vi "FTW-SyncServer-Reply.vi"(0 "FTW Synchronous Server":refnum<data-value>, 5 "Response":string, 7 "Send Timeout":i32 format="%dmsec", 11 "error in":errorcluster) -> (4 "FTW Synchronous Server out":refnum<data-value>, 15 "error out":errorcluster)   [LabVIEW 2014]
uses:
  core/FTW-SyncServer-Core-Type.ctl
  error/FTW-ERR-ThrowGenericError.vi
  error/FTW-ERR-ThrowError.vi
  error/FTW-ERR-CallChain.vi
  string/FTW-STR-ReplaceWhitespace.vi
panel:
  # "Inputs"
  # "Outputs"
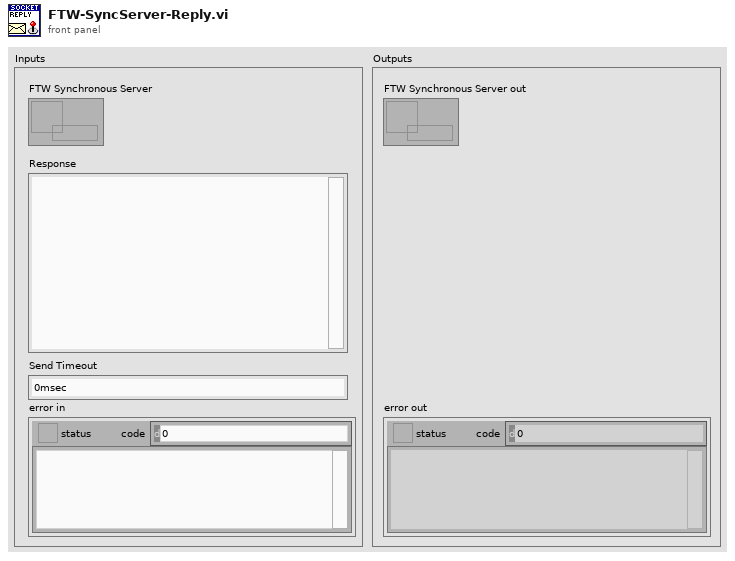
[diagram p1: front panel]
types:
  T1 = typedef "FTW-SyncServer-Core-Type.ctl" = cluster{"Socket":i64}
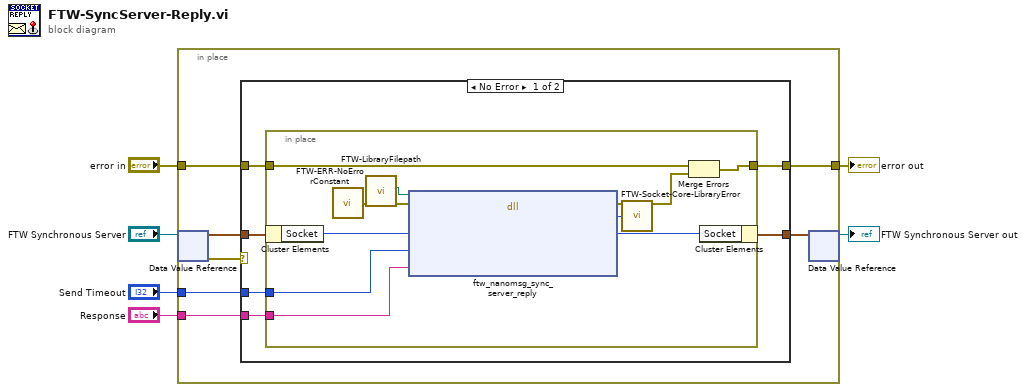
[diagram p0: block diagram]
diagram:
  n1 = in-place {
    in-place-border: "error in" -> [w13]
    in-place-border: [w12] -> w2
    in-place-border: "Send Timeout" -> [w11]
    in-place-border: "Response" -> [w10]
    n2 = in-place-dvr #1("FTW Synchronous Server") -> (w9:T1, w7:errorcluster)
    n3 = case shown="No Error" w7 {
      tunnel: w13 -> [w19 w33]
      tunnel: [w18 w33] -> w12
      tunnel: w11 -> [w17 _]
      tunnel: w10 -> [w16 _]
      tunnel: w9 -> [w15 w32]
      tunnel: [w14 w32] -> w8
      frame No Error {
        n4 = in-place {
          in-place-border: w19 -> [w22]
          in-place-border: [w24] -> w18
          in-place-border: w17 -> [w28]
          in-place-border: w16 -> [w21]
          n5 = in-place-cluster #2(w15) -> ("Socket"=w26:i64)
          n6 = call "FTW-ERR-NoErrorConstant.vi"() -> ("no error"=w20:errorcluster)
          n7 = call "FTW-LibraryFilepath.vi"("error in"=w20) -> ("error out"=w29:errorcluster, "Library Filepath"=w30:path)  [unwired: 8 in, 1 out]
          n8 = dll-call lib="?" fn="ftw_nanomsg_sync_server_reply"(path in=w30, error in=w29, "Socket Handle"=w26, "Send Timeout"=w28, "Response"=w21) -> (error out=w31:errorcluster, "Return Value"=w27:i64, "Socket Handle"=w25:i64)  [unwired: 3 in, 1 out]
          n9 = call "FTW-Socket-Core-LibraryError.vi"("error in"=w31, "Return Value"=w27) -> ("error out"=w23:errorcluster)  [unwired: 13 in]
          n10 = Merge Errors(w22, w23) -> (w24:errorcluster)
          n11 = in-place-cluster #2("Socket"=w25) -> (w14:T1)
        }
      }
      frame Error {
      }
    }
    n12 = in-place-dvr #1(w8) -> (→"FTW Synchronous Server out":refnum<data-value>)  [unwired: 1 out]
  }
  "error out" <- w2
